vi "Set Plot Visibility (XYGraph).vi"(8 "error in (no error)":errorcluster, 10 "Plot.Visible?":bool[](array[boolean]), 11 "XYGraph in":refnum<vi>) -> (0 "error out":errorcluster)   [LabVIEW 2019, in "Instrument.Lockin.lvlib" / "Instrument UI.Lockin.lvclass"]
uses:
  Instrument UI.Lockin.lvclass
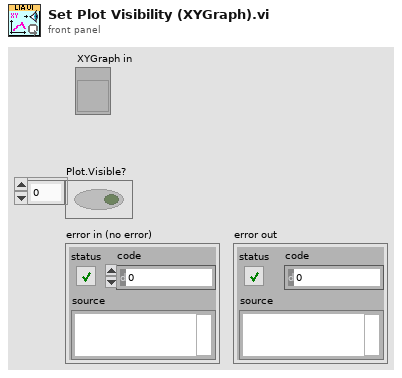
[diagram p1: front panel]
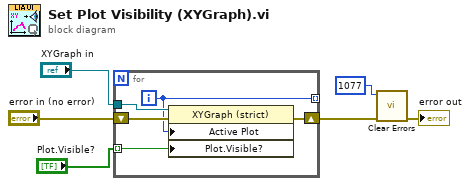
[diagram p0: block diagram]
diagram:
  n1 = for {
    tunnel: "XYGraph in" -> [w11]
    tunnel: [w7] -> _ mode=indexing
    tunnel: "Plot.Visible?" -> [w9] mode=indexing
    shift-right: [w8] -> w2
    shift-left: "error in (no error)" -> [w10]
    i -> [w7]
    n2 = property on="Property Node" class="XYGraph (strict)"(reference=w11, error in=w10, "Active Plot"=w7, "Plot.Visible?"=w9) -> (error out=w8:errorcluster)  [unwired: 1 out]
  }
  n3 = call <vilib>:"Clear Errors.vi"("error in (no error)"=w2, "specific error code to clear (0: all)"=1077) -> ("error out"=→"error out":errorcluster)  [unwired: 4 in, 1 out]
